vi "DAQNavi Read (Counter Pulse Width 1Chan 1Samp).vi"(8 "error in (no error)":errorcluster, 10 "timeout":dbl=10.0, 11 "task in":i32) -> (0 "error out":errorcluster, 2 "data":cluster{"high period":dbl, "low period":dbl}, 3 "task out":i32)   [LabVIEW 2020]
uses:
  DAQNavi_LV.dll
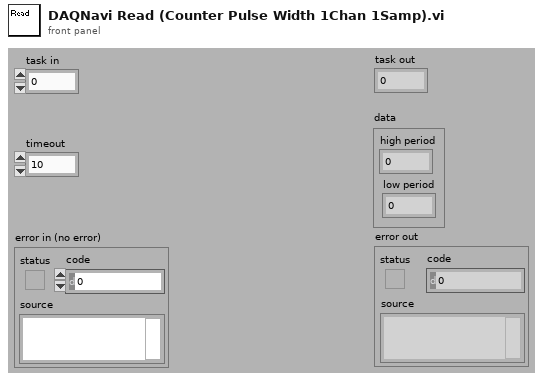
[diagram p1: front panel]
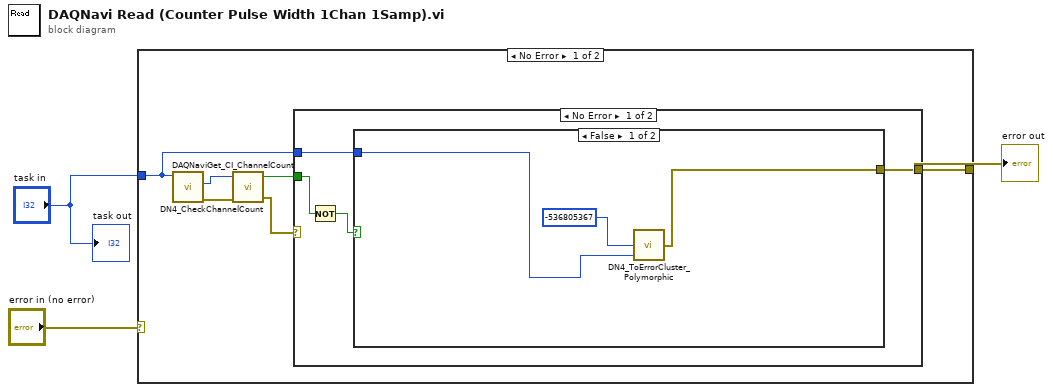
[diagram p0: block diagram]
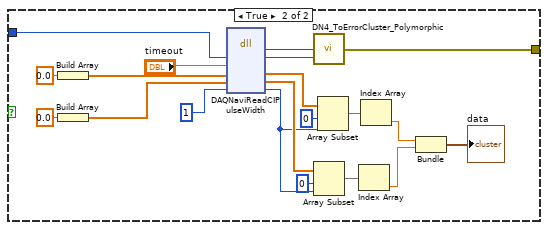
[diagram p2: hidden frame]
diagram:
  n1 = case shown="No Error" "error in (no error)" {
    selector: "error in (no error)" -> [_ w38]
    tunnel: "task in" -> [w4 _]
    tunnel: [w9 w38] -> w1
    frame No Error {
      n2 = call "DAQNaviGet_CI_ChannelCount.vi"("task in"=w4) -> ("error out"=w8:errorcluster, "channel count"=w7:i32)  [unwired: 1 in, 8 out]
      n3 = call "DN4_CheckChannelCount.vi"("error out"=w8, "channel count"=w7) -> ("error IO"=w6:errorcluster, "greater than 1?"=w5:bool)  [unwired: 2 out]
      n4 = case shown="No Error" w6 {
        selector: w6 -> [_ w37]
        tunnel: [w13 w37] -> w9
        tunnel: w5 -> [w11 _]
        tunnel: w4 -> [w10 _]
        frame No Error {
          n5 = Not(x=w11) -> (.not. x?=w12:bool)
          n6 = case shown="False" w12 {
            tunnel: [w14 w36] -> w13
            tunnel: w10 -> [w16 w17]
            frame False {
              n7 = call "DN4_ToErrorCluster_Polymorphic.vi"("task id"=w16, "error code"=-536805367) -> ("error out"=w14:errorcluster)  [unwired: 3 out]
            }
            frame True {
              n8 = Build Array(0.0 ("element")) -> (w31:dbl[])
              n9 = Build Array(0.0 ("element")) -> (w27:dbl[])
              n10 = dll-call lib="DAQNavi_LV.dll" fn="DAQNaviReadCIPulseWidth"("taskID"=w17, "timeout"="timeout", "hiPeriod"=w31, "loPeriod"=w27, "samples"=u32 1) -> ("return type"=w34:i32, "taskID"=w18:i32, "hiPeriod"=w22:dbl[], "loPeriod"=w26:dbl[], "samples"=w23:u32)  [unwired: 4 in, 2 out]
              n11 = call "DN4_ToErrorCluster_Polymorphic.vi"("task id"=w18, "error code"=w34) -> ("error out"=w36:errorcluster)  [unwired: 3 out]
              n12 = Array Subset(array=w26, index=0, length=w23) -> (w29:dbl[])
              n13 = Array Subset(array=w22, index=0, length=w23) -> (w24:dbl[])
              n14 = Index Array(array=w29) -> (element=w20:dbl)  [unwired: 1 in]
              n15 = Index Array(array=w24) -> (element=w21:dbl)  [unwired: 1 in]
              n16 = Bundle(w21, w20) -> (→"data":cluster{dbl, dbl})  [unwired: 1 out]
            }
          }
        }
        frame Error {
        }
      }
    }
    frame Error {
    }
  }
  "error out" <- w1
  "task out" <- "task in"
